vi "DatSaveParams.vi"(6 "error in (no error)":errorcluster, 7 "Values":dbl[](array[numeric])=[1.0, 2.0], 8 "Names":string[](array[string])=["par1", "par2"], 9 "tracename":string="F:\\2017 10 06\\current vi's\\Data\\data_025.tdms: 2") -> (0 "error out":errorcluster, 3 "tracename out":string)   [LabVIEW 2018]
uses:
  <vilib>/Utility/file.llb/Write To Spreadsheet File (string).vi
  <vilib>/Utility/file.llb/Read From Spreadsheet File (string).vi
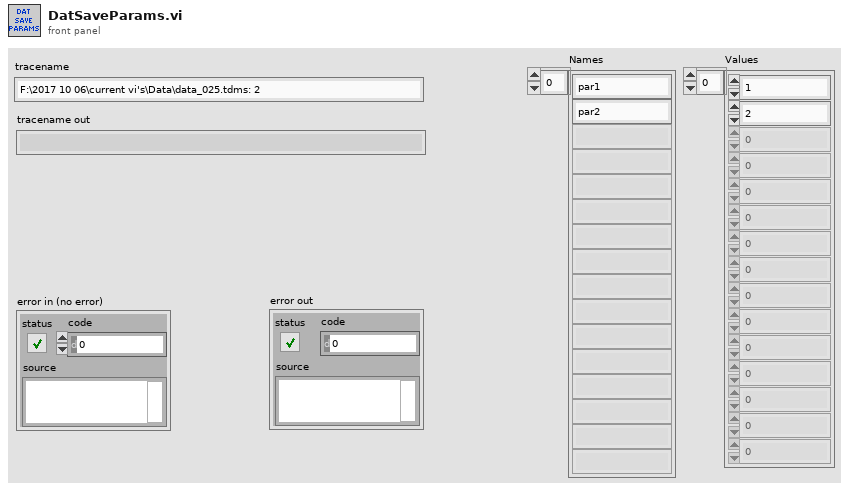
[diagram p1: front panel]
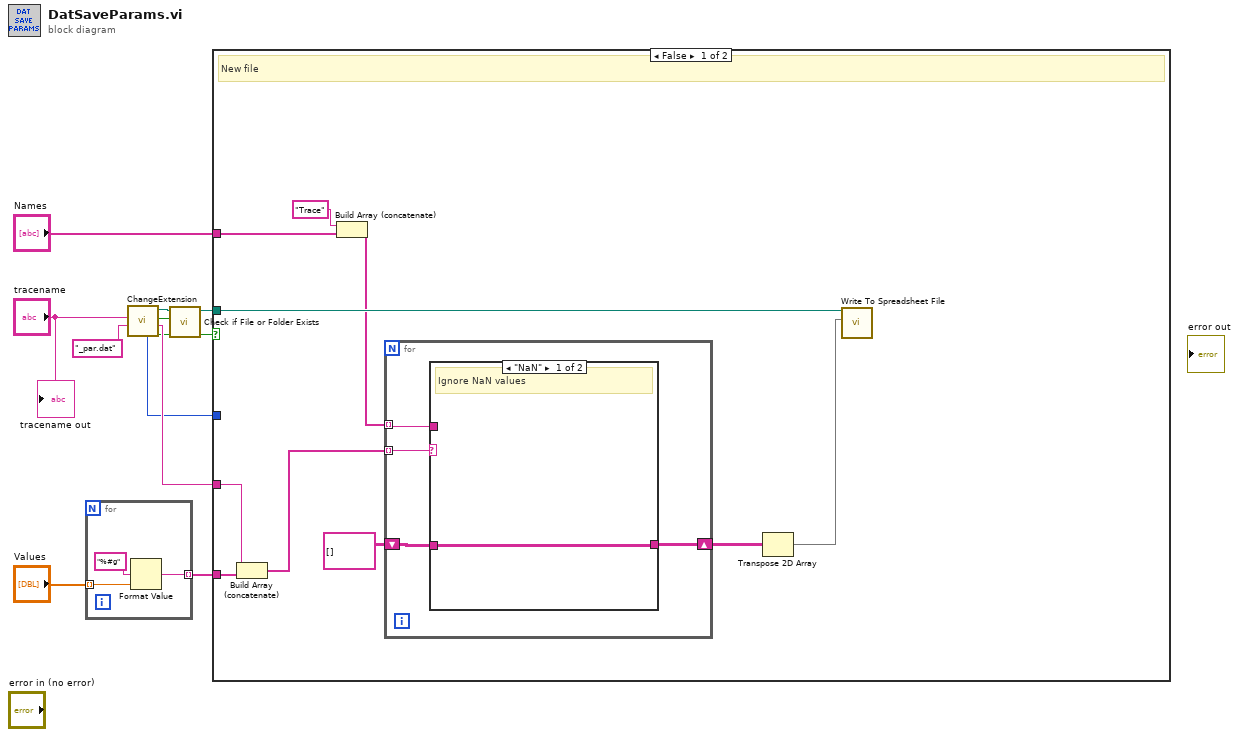
[diagram p0: block diagram]
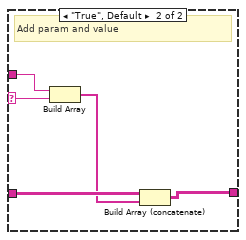
[diagram p2: hidden frame]
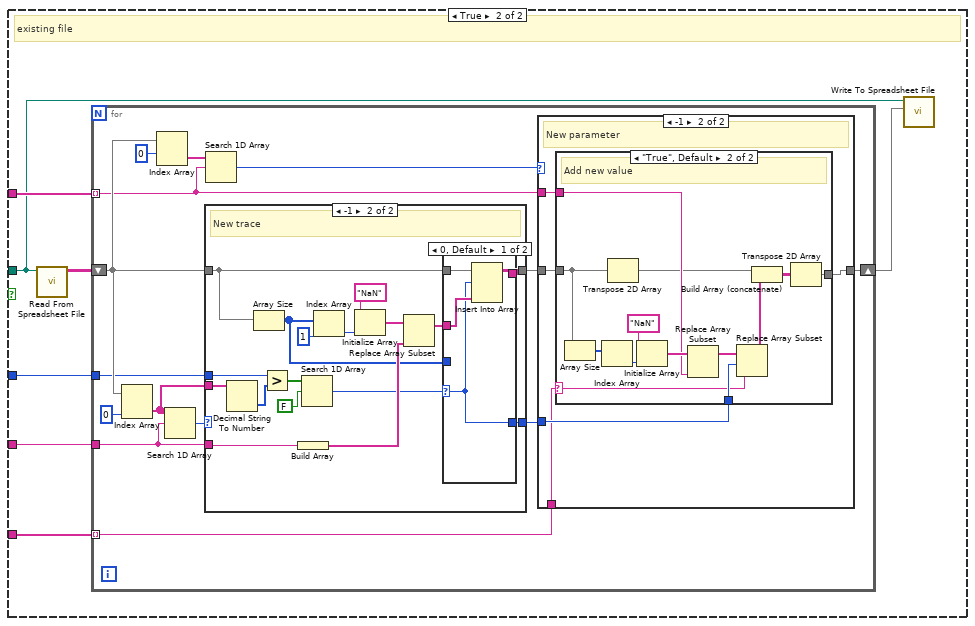
[diagram p3: hidden frame]
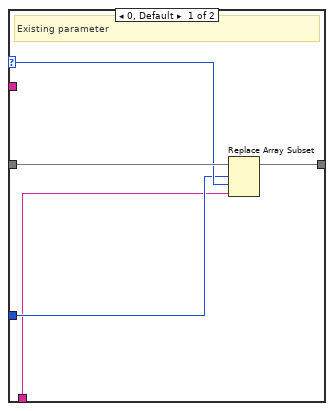
[diagram p4: hidden frame]
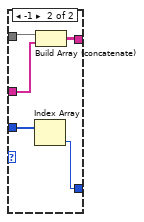
[diagram p7: hidden frame]
diagram:
  n1 = for {
    tunnel: "Values" -> [w13] mode=indexing
    tunnel: [w11] -> w2 mode=indexing
    n2 = Format Value(format string="%#g", value (0)=w13) -> (output string=w11:string)  [unwired: 1 in]
  }
  n3 = call "ChangeExtension.vi"("extension"="_par.dat", "file in"="tracename") -> (1:"Tracenr"=w5:string, "Path out"=w7:path, 4:"Tracenr"=w1:i32)  [unwired: 3 in, 2 out]
  n4 = call <vilib>:"Check if File or Folder Exists.vi"("path"=w7) -> ("file or folder exists?"=w4:bool, "dup path"=w6:path)  [unwired: 8 in, 1 out]
  n5 = case shown="False" w4 {
    tunnel: "Names" -> [w22 w40]
    tunnel: w6 -> [w23 w34]
    tunnel: w5 -> [w20 w39]
    tunnel: w2 -> [w17 w38]
    tunnel: w1 -> [_ w36]
    frame False {
      # "New file"
      n6 = Build Array (concatenate)(w20, w17) -> (w19:string[])
      n7 = Build Array (concatenate)("Trace" ("trace name"), w22) -> (w21:string[])
      n8 = for {
        tunnel: w21 -> [w27] mode=indexing
        tunnel: w19 -> [w26] mode=indexing
        shift-right: [w24] -> w15
        shift-left: string[][] [] -> [w25]
        n9 = case shown="\"NaN\"" w26 {
          selector: w26 -> [_ w29]
          tunnel: w27 -> [_ w33]
          tunnel: w25 -> [w28 w32]
          tunnel: [w28 w30] -> w24
          frame "NaN" {
            # "Ignore NaN values"
          }
          frame "True", Default {
            # "Add param and value"
            n10 = Build Array(w33, w29) -> (w31:string[])
            n11 = Build Array (concatenate)(w32, w31) -> (w30:string[][])
          }
        }
      }
      n12 = Transpose 2D Array(2D array=w15) -> (transposed array=w14:string[][])
      n13 = call-poly <vilib>:"Write To Spreadsheet File.vi"("2D data"=w14, "file path (dialog if empty)"=w23) -> ()  [unwired: 6 in, 1 out]
    }
    frame True {
      # "existing file"
      n14 = call-poly <vilib>:"Read From Spreadsheet File.vi"("file path (dialog if empty)"=w34) -> ("all rows"=w37:string[][])  [unwired: 6 in, 4 out]
      n15 = for {
        tunnel: w40 -> [w47] mode=indexing
        tunnel: w39 -> [w52]
        shift-right: [w48] -> w35
        shift-left: w37 -> [w50]
        tunnel: w38 -> [w42] mode=indexing
        tunnel: w36 -> [w45]
        n16 = Index Array(array=w50, index (col)=0 ("disabled index (col)")) -> (element=w46:string[])  [unwired: 1 in]
        n17 = Index Array(array=w50, index (row)=0) -> (element=w49:string[])  [unwired: 1 in]
        n18 = Search 1D Array(1D array=w46, element=w52) -> (index of element=w53:i32)  [unwired: 1 in]
        n19 = case shown="-1" w53 {
          selector: w53 -> [w79 _]
          tunnel: w50 -> [w80 w87]
          tunnel: w52 -> [_ w94]
          tunnel: [w80 w85] -> w44
          tunnel: [w79 w83] -> w41
          tunnel: w46 -> [_ w92]
          tunnel: w45 -> [_ w91]
          frame 0, Default {
            # "Existing trace"
          }
          frame -1 {
            # "New trace"
            n20 = Decimal String To Number(string=w92) -> (number=w90:i32[])  [unwired: 2 in, 1 out]
            n21 = Array Size(array=w87) -> (size(s)=w81:i32[])
            n22 = Greater?(x=w91, y=w90) -> (0:w89:bool[])
            n23 = Build Array(w94) -> (w93:string[])
            n24 = Search 1D Array(1D array=w89, element=FALSE) -> (index of element=w84:i32)  [unwired: 1 in]
            n25 = Index Array(array=w81, index=1) -> (element=w82:i32)
            n26 = Initialize Array("NaN" ("F-format string"), w82) -> (w95:string[])
            n27 = Replace Array Subset(array=w95, new element=w93) -> (w86:string[])  [unwired: 1 in]
            n28 = case shown="0, Default" w84 {
              selector: w84 -> [w98 _]
              tunnel: w87 -> [w101 w106]
              tunnel: w86 -> [w100 w105]
              tunnel: [w99 w104] -> w85
              tunnel: [w98 w102] -> w83
              tunnel: w81 -> [_ w103]
              frame 0, Default {
                n29 = Insert Into Array(array=w101, index (row)=w98, new element=w100) -> (w99:string[][])  [unwired: 1 in]
              }
              frame -1 {
                n30 = Index Array(array=w103) -> (element=w102:i32)  [unwired: 1 in]
                n31 = Build Array (concatenate)(w106, w105) -> (w104:string[][])
              }
            }
          }
        }
        n32 = Search 1D Array(1D array=w49, element=w47) -> (index of element=w43:i32)  [unwired: 1 in]
        n33 = case shown="-1" w43 {
          selector: w43 -> [w58 _]
          tunnel: w44 -> [w59 w62]
          tunnel: w41 -> [w57 w63]
          tunnel: w42 -> [w56 w60]
          tunnel: [w55 w61] -> w48
          tunnel: w47 -> [_ w64]
          frame 0, Default {
            # "Existing parameter"
            n34 = Replace Array Subset(array=w59, new element=w56, index (row)=w57, index (col)=w58) -> (w55:string[][])
          }
          frame -1 {
            # "New parameter"
            n35 = case shown="\"True\", Default" w60 {
              selector: w60 -> [_ w66]
              tunnel: w64 -> [_ w74]
              tunnel: w63 -> [_ w72]
              tunnel: w62 -> [w65 w71]
              tunnel: [w65 w67] -> w61
              frame "NaN" {
                # "No need to add"
              }
              frame "True", Default {
                # "Add new value"
                n36 = Array Size(array=w71) -> (size(s)=w78:i32[])
                n37 = Index Array(array=w78) -> (element=w77:i32)  [unwired: 1 in]
                n38 = Transpose 2D Array(2D array=w71) -> (transposed array=w70:string[][])
                n39 = Initialize Array("NaN" ("F-format string"), w77) -> (w75:string[])
                n40 = Replace Array Subset(array=w75, new element=w74) -> (w73:string[])  [unwired: 1 in]
                n41 = Replace Array Subset(array=w73, new element=w66, index=w72) -> (w69:string[])
                n42 = Build Array (concatenate)(w70, w69) -> (w68:string[][])
                n43 = Transpose 2D Array(2D array=w68) -> (transposed array=w67:string[][])
              }
            }
          }
        }
      }
      n44 = call-poly <vilib>:"Write To Spreadsheet File.vi"("2D data"=w35, "file path (dialog if empty)"=w34) -> ()  [unwired: 6 in, 1 out]
    }
  }
  "tracename out" <- "tracename"
